vi "KE2260B Output Protection Status.vi"(8 "error in (no error)":errorcluster, 11 "VISA resource name":refnum<visa-resource-name>) -> (0 "error out":errorcluster, 1 "OCP Tripped?":bool, 2 "OVP Tripped?":bool, 3 "VISA resource name out":refnum<visa-resource-name>)   [LabVIEW 2009, in "Keithley 2260B.lvlib"]
doc: "Returns over voltage protection (OVP) and over current protection (OCP) status."
uses:
  <instrlib>/Keithley 2260B/Keithley 2260B.lvlib
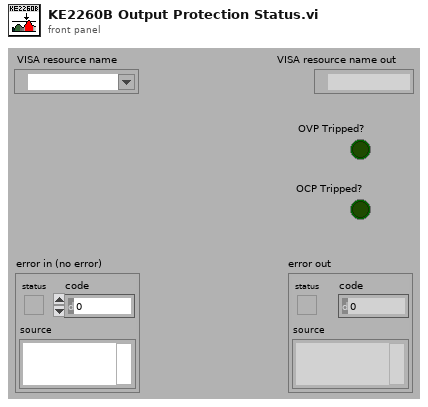
[diagram p1: front panel]
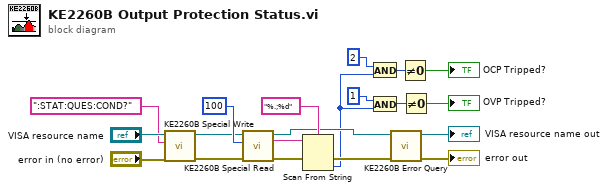
[diagram p0: block diagram]
diagram:
  n1 = call <instrlib>:"KE2260B Special Write.vi"("error in (no error)"="error in (no error)", "Write Buffer (\"\")"=":STAT:QUES:COND?" ("write buffer"), "VISA session"="VISA resource name") -> ("error out"=w5:errorcluster, "dup VISA session"=w1:refnum<visa-resource-name>)  [unwired: 6 in, 1 out]
  n2 = call <instrlib>:"KE2260B Special Read.vi"("error in (no error)"=w5, "byte count"=u32 100, "VISA session"=w1) -> ("error out"=w15:errorcluster, "read buffer"=w17:string, "dup VISA session"=w13:refnum<visa-resource-name>)  [unwired: 5 in, 1 out]
  n3 = Scan From String(format string="%.;%d", input string=w17, error in=w15) -> (error out=w14:errorcluster, output 1=w9:i32)  [unwired: 2 in, 2 out]
  n4 = And(x=2, y=w9) -> (x .and. y?=w11:i32)
  n5 = And(x=1, y=w9) -> (x .and. y?=w7:i32)
  n6 = call <instrlib>:"KE2260B Error Query.vi"("error in (no error)"=w14, "VISA resource name"=w13) -> ("error out"=→"error out":errorcluster, "VISA resource name out"=→"VISA resource name out":refnum<visa-resource-name>)  [unwired: 6 in, 2 out]
  n7 = Not Equal To 0?(x=w11) -> (x != 0?=→"OCP Tripped?":bool)
  n8 = Not Equal To 0?(x=w7) -> (x != 0?=→"OVP Tripped?":bool)
